vi "ReceiveDataFromWindow(SubVI).vi"(4 "Boolean in":refnum<vi>, 5 "queue in":refnum<queue>, 6 "CmbBox Refnum":refnum<vi>, 7 "STM Graph":T1 {"Lines"."Color" format="%x"}, 8 "Error In":errorcluster, 9 "XY Graph":refnum<vi>, 10 "Lines":refnum<vi>, 11 "Clust Refnum":refnum<vi>) -> (0 "Error Out":errorcluster, 3 "queue out":refnum<queue>)   [LabVIEW 2018]
uses:
  STM/Grafic/MOKO_Grafic_STM.ctl
  STM/Grafic/MOKO_Grafic_ITEM.ctl
  CTL/STM GRAPH.ctl
  CTL/Graph settings.ctl
  CTL/Line.ctl
  Windows/Settings/View.ctl
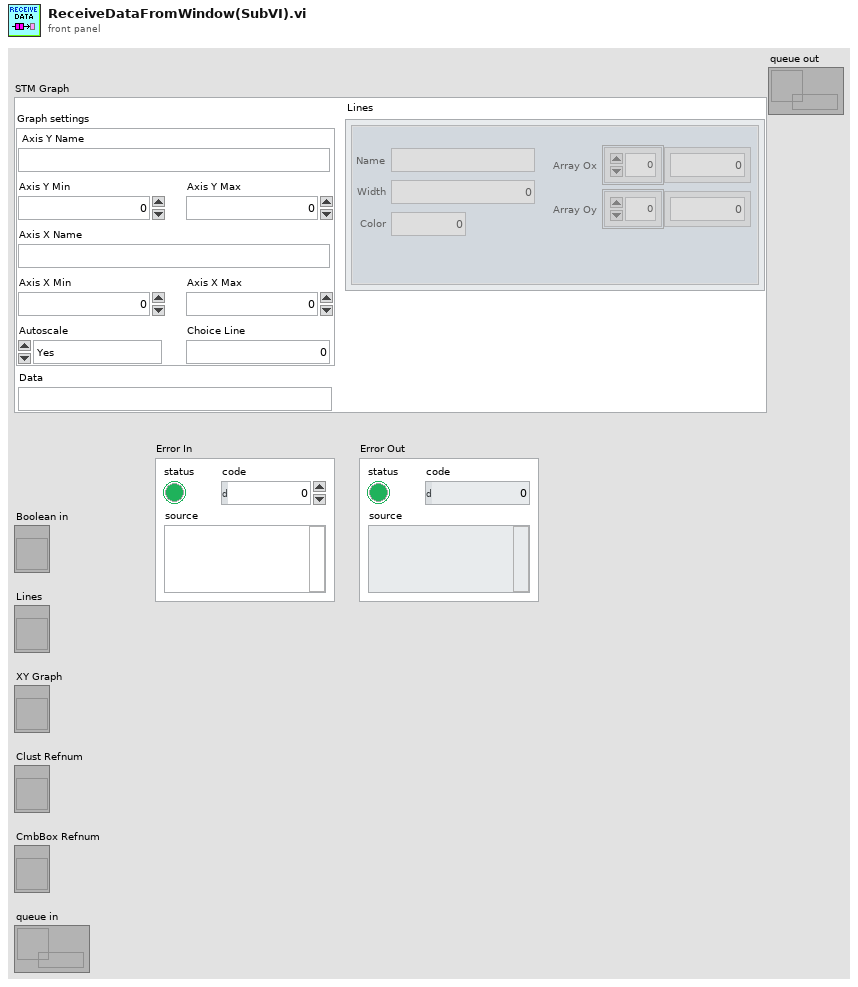
[diagram p1: front panel]
types:
  T1 = typedef "STM GRAPH.ctl" = cluster{"Graph settings":T2, "Lines":T3[], "Data":string}
  T2 = typedef "Graph settings.ctl" = cluster{"Axis X Min":dbl, "Axis X Name":string, "Axis X Max":dbl, "Axis Y Min":dbl, " Axis Y Name":string, "Axis Y Max":dbl, "Autoscale":enum16{"Yes", "No", "Only Oy", "Only Ox"}, "Choice Line":dbl}
  T3 = typedef "Line.ctl" = cluster{"Width":dbl, "Color":i64, "Array Oy":dbl[], "Array Ox":dbl[], "Name":string, "Plot Visible":T4}
  T4 = typedef "View.ctl" = bool
  T5 = typedef "MOKO_Grafic_STM.ctl" = cluster{"main stm":T6, "STM Graph":T1}
  T6 = typedef "MOKO_Grafic_ITEM.ctl" = enum16{"idle", "init", "_____ LINE _____ ", "_____ WINDOW _____ ", "_____ BUTTONS _____ ", "_____ GRAPH _____ ", "Legend", "Write Graph", "Clear Graph", "close", "Screenshot", "Add Line", "Change Line", "Graph Settings", "Delete Line", "Autoscale", "Hide Line", "Show Line", "Send Data", "Receive Data"}
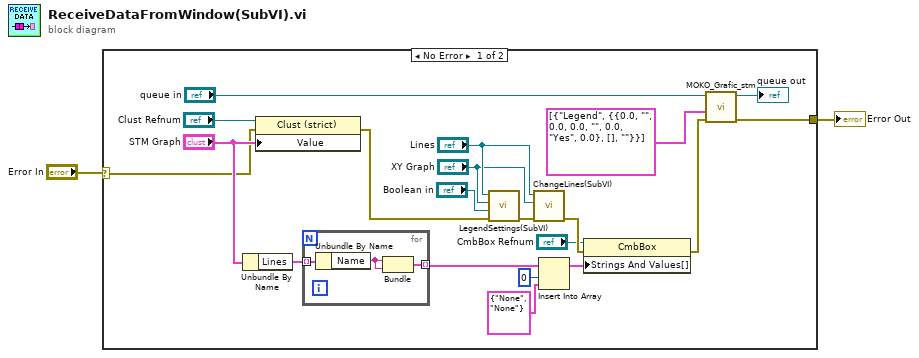
[diagram p0: block diagram]
diagram:
  n1 = case shown="No Error" "Error In" {
    selector: "Error In" -> [w4 w26]
    tunnel: [w3 w26] -> w1
    frame No Error {
      n2 = Unbundle By Name("STM Graph") -> ("Lines"=w15:T3[])
      n3 = property on="Property Node" class="Clust (strict)"(reference="Clust Refnum", error in=w4, "Value"="STM Graph") -> (error out=w11:errorcluster)  [unwired: 1 out]
      n4 = for {
        tunnel: w15 -> [w25] mode=indexing
        tunnel: [w23] -> w14 mode=indexing
        n5 = Unbundle By Name(w25) -> ("Name"=w24:string)
        n6 = Bundle("Name"=w24, "Name"=w24) -> (w23:cluster{"Name":string, "Name":string})  [unwired: 1 in]
      }
      n7 = call "LegendSettings(SubVI).vi"("Error In"=w11, "Legend"="Boolean in", "XYGraph Refnum"="XY Graph", "Arr Refnum"="Lines") -> ("Error Out"=w10:errorcluster)  [unwired: 7 in]
      n8 = call "ChangeLines(SubVI).vi"("Error In"=w10, "XYGraph Refnum"="XY Graph", "Arr Refnum"="Lines") -> ("Error Out"=w21:errorcluster)  [unwired: 8 in]
      n9 = Insert Into Array(array=w14, index=0, new element=cluster{"Name":string, "Name":string} {"Name"="None", "Name"="None"} ("new element/subarray")) -> (w17:cluster{"Name":string, "Name":string}[])
      n10 = property on="Property Node" class="CmbBox"(reference="CmbBox Refnum", error in=w21, "Strings And Values[]"=w17) -> (error out=w22:errorcluster)  [unwired: 1 out]
      n11 = call "MOKO_Grafic_stm.vi"("error in"=w22, "StateMachineSteps"=T5[] [{"main stm"=enum."Legend", "STM Graph"={"Graph settings"={"Axis X Min"=0.0, "Axis X Name"="", "Axis X Max"=0.0, "Axis Y Min"=0.0, " Axis Y Name"="", "Axis Y Max"=0.0, "Autoscale"=enum."Yes", "Choice Line"=0.0}, "Lines"=[], "Data"=""}}], "queue in"="queue in") -> ("error out"=w3:errorcluster, "queue out"=→"queue out":refnum<queue>)  [unwired: 7 in]
    }
    frame Error {
    }
  }
  "Error Out" <- w1
